vi "SwerveHeadingLock2.vi"(3 "Driver Rotation Joystick":dbl, 6 "PID Tuning Parameters":T2={"Kp"=0.0, "Ki"=0.0, "Kd"=0.0, "N-Diff"=10, "N-Int"=10, "Int Error Window"=30.0, "Max Ouput"=1.0, "Min Output"=-1.0} {"Int Error Window" min=0.0; "N-Int" min=2; "N-Diff" min=2; "Kd" min=0.0; "Ki" min=0.0; "Kp" min=0.0}, 10 "Heading Lock Strafe Deadband (ft/s)":dbl, 12 "External Disables":bool) -> (14 "Controller Summary":T1(graph), 17 "Joystick Rotation":dbl, 19 "Heading Lock":bool)   [LabVIEW 2019]
uses:
  sensors.vi
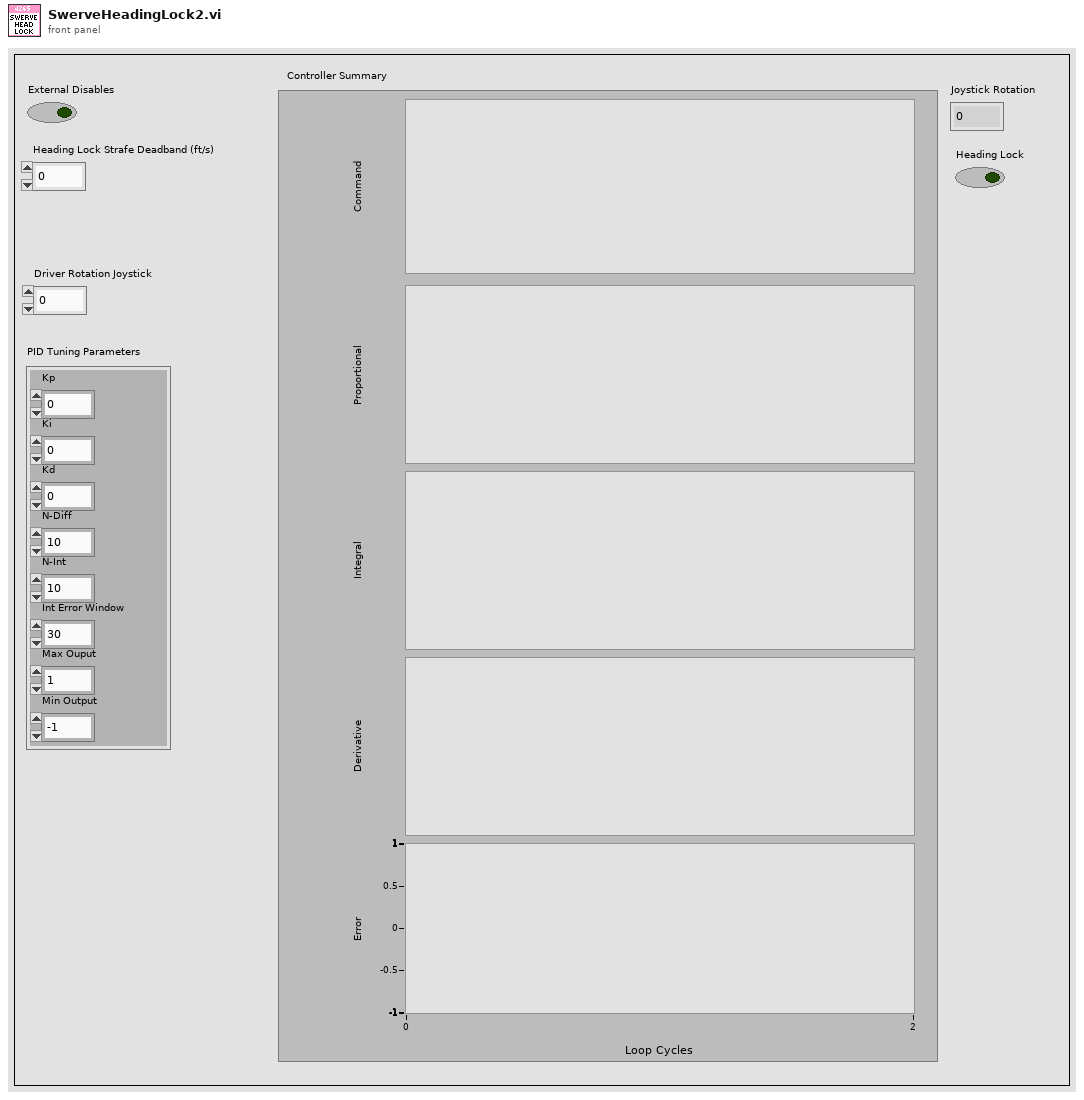
[diagram p1: front panel]
types:
  T1 = cluster{"Command":dbl, "Proportional":dbl, "Integral":dbl, "Derivative":dbl, "Goal":dbl}
  T2 = cluster{"Kp":dbl, "Ki":dbl, "Kd":dbl, "N-Diff":i32, "N-Int":i32, "Int Error Window":dbl, "Max Ouput":dbl, "Min Output":dbl}
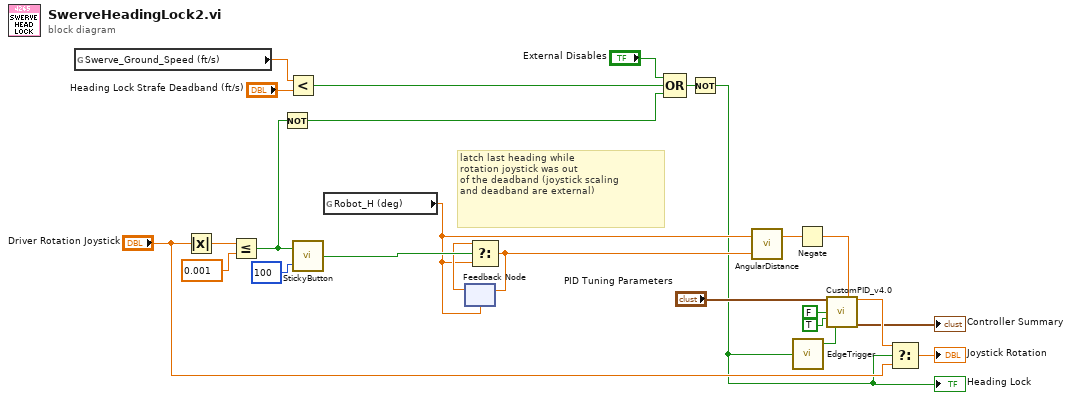
[diagram p0: block diagram]
diagram:
  # "latch last heading while\nrotation joystick was out \nof the deadband (joystick scaling \nand deadband are external)"
  n1 = global read "sensors.vi" "Swerve_Ground_Speed (ft/s)"() -> (w1:dbl)
  n2 = Absolute Value(x="Driver Rotation Joystick") -> (abs(x)=w19:dbl)
  n3 = Less Or Equal?(x=w19, y=0.001) -> (x <= y?=w7:bool)
  n4 = Not(x=w7) -> (.not. x?=w6:bool)
  n5 = Less?(x=w1, y="Heading Lock Strafe Deadband (ft/s)") -> (x < y?=w2:bool)
  n6 = call "StickyButton.vi"("Time threshold (ms)"=u32 100 ("y"), "Button Input"=w7) -> ("Sticky Button"=w10:bool)
  n7 = global read "sensors.vi" "Robot_H (deg)"() -> (w8:dbl)
  n8 = feedback #1(w8) -> (w9:dbl)
  n9 = Select(t=w9, s=w10, f=w8) -> (s? t:f=w20:dbl)
  n10 = feedback-in #1(w20) -> ()
  n11 = Compound Arithmetic op=OR("External Disables", w2, w6) -> (w5:bool)
  n12 = Not(x=w5) -> (.not. x?=w4:bool)
  "Heading Lock" <- w4
  n13 = call "AngularDistance.vi"("Goal Angle (deg) [0,360]"=w20, "Current Angle (deg) [-Inf,+Inf]"=w8) -> ("Signed Angular Distance (deg) [-180,+180]"=w18:dbl)  [unwired: 1 out]
  n14 = call "EdgeTrigger.vi"("Input Signal"=w4) -> ("Rising Edge Trigger"=w23:bool)  [unwired: 2 out]
  n15 = Negate(x=w18) -> (-x=w21:dbl)
  n16 = call "CustomPID_v4.0.vi"("PID Tuning Parameters"="PID Tuning Parameters", "Custom Error Calculation"=w21, "Reset on Goal Change ?"=FALSE, "Use Custom Error Calculation ?"=TRUE, "Reinit"=w23) -> ("Command"=w17:dbl, "Controller Summary"=→"Controller Summary":T1)  [unwired: 7 in, 2 out]
  n17 = Select(t=w17, s=w4, f="Driver Rotation Joystick") -> (s? t:f=→"Joystick Rotation":dbl)
